vi "archivoAdiciónTexto.vi"() -> ()   [LabVIEW 2011]
panel:
  out "Array":dbl[](array[numeric])
  # "programa para adicionar datos a un archio de texto"
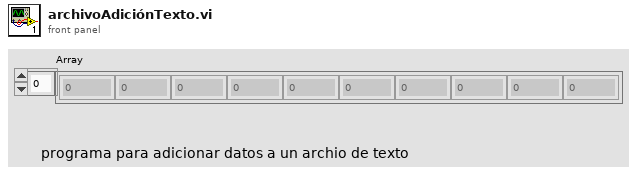
[diagram p1: front panel]
types:
  T1 = enum16{"open", "replace", "create", "open or create", "replace or create", "replace or create with confirmation"}
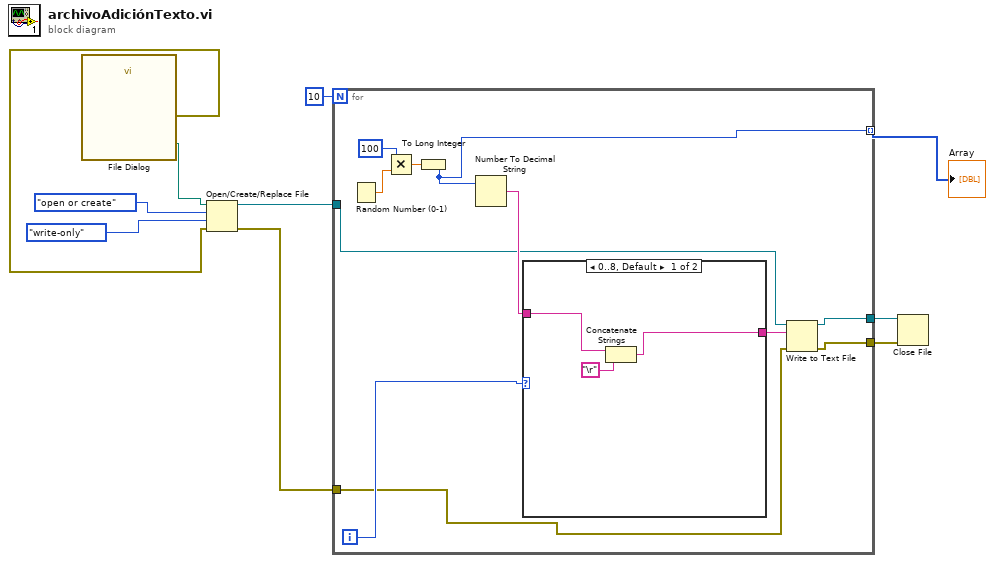
[diagram p0: block diagram]
diagram:
  n1 = call "File Dialog"() -> ("selected path"=w10:path, "error out"=w7:errorcluster)  [unwired: 12 in, 2 out]
  n2 = Open/Create/Replace File(file path (use dialog)=w10, error in=w7, operation (0:open)=T1."open or create", access (0:read/write)=enum16{"read/write", "read-only", "write-only"}."write-only") -> (refnum out=w4:refnum<file>, error out=w3:errorcluster)  [unwired: 2 in, 1 out]
  n3 = for {
    N: 10 -> [_]
    tunnel: [w17] -> w5 mode=indexing
    tunnel: w4 -> [w14]
    tunnel: w3 -> [w13]
    tunnel: [w12] -> w2
    tunnel: [w11] -> w1
    i -> [w18]
    n4 = Random Number (0-1)() -> (number: 0 to 1=w20:dbl)
    n5 = Multiply(x=100, y=w20) -> (x*y=w19:dbl)
    n6 = To Long Integer(number=w19) -> (32bit integer=w17:i32)
    n7 = Number To Decimal String(number=w17) -> (decimal integer string=w16:string)  [unwired: 1 in]
    n8 = case shown="0..8, Default" w18 {
      tunnel: w16 -> [w24 w25]
      tunnel: [w22 w25] -> w15
      frame 0..8, Default {
        n9 = Concatenate Strings "Concatenate Strings"(w24, "\r") -> (w22:string)
      }
      frame 9 {
      }
    }
    n10 = Write to Text File(file (use dialog)=w14, text=w15, error in=w13) -> (refnum out=w12:refnum<file>, error out=w11:errorcluster)  [unwired: 1 in, 1 out]
  }
  "Array" <- w5
  n11 = Close File(refnum=w2, error in=w1) -> ()  [unwired: 2 out]
